vi "DMS_Multiplexer_Final.vi"() -> ()   [LabVIEW 2011]
uses:
  <vilib>/Instr/_visa.llb/VISA Configure Serial Port (Instr).vi
panel:
  out "error out":errorcluster
  in  "Dwell Time(s)":i32=20
  in  "No of Channels":i32=4
  in  "VISA resource name":refnum<visa-resource-name>="COM7"
  in  "Port B Read command\n(ASCII 'A'/41H)":string="Aÿ"
  out "USB Output String\n     (Bits 1-4)":string
  out "USB Port read status\n (Bits 8-5 = DIO, Bits 4-1 = Relays)":string
  out "Number":u32 format="%.0x"
  in  "Port B (Bits 1-8) Direction command\n (ASCII 'B'/42H)\n(0=output/1=input)":string="Bð"
  in  "Delay period \n(between channel activation)":dbl=20.0
  in  "Quit":bool
  # "USB4Mx (LV7.1 - Visa serial vi's)\n(8 bit (Port B) 4 output & 4 input channels)"
  # "Port Configuration/\nInitialisation characters"
  # "Relay control (Channels 1-4)"
  # "Port B Write command\n(ASCII 'C'/43H)"
  # "Voltage input channel status (Channels 8-5)"
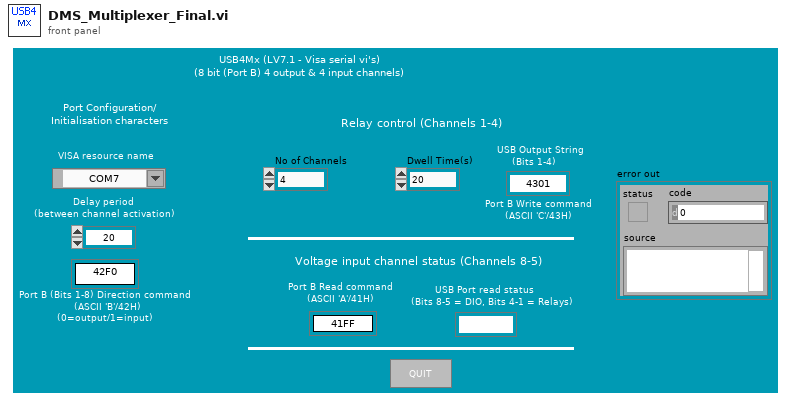
[diagram p1: front panel]
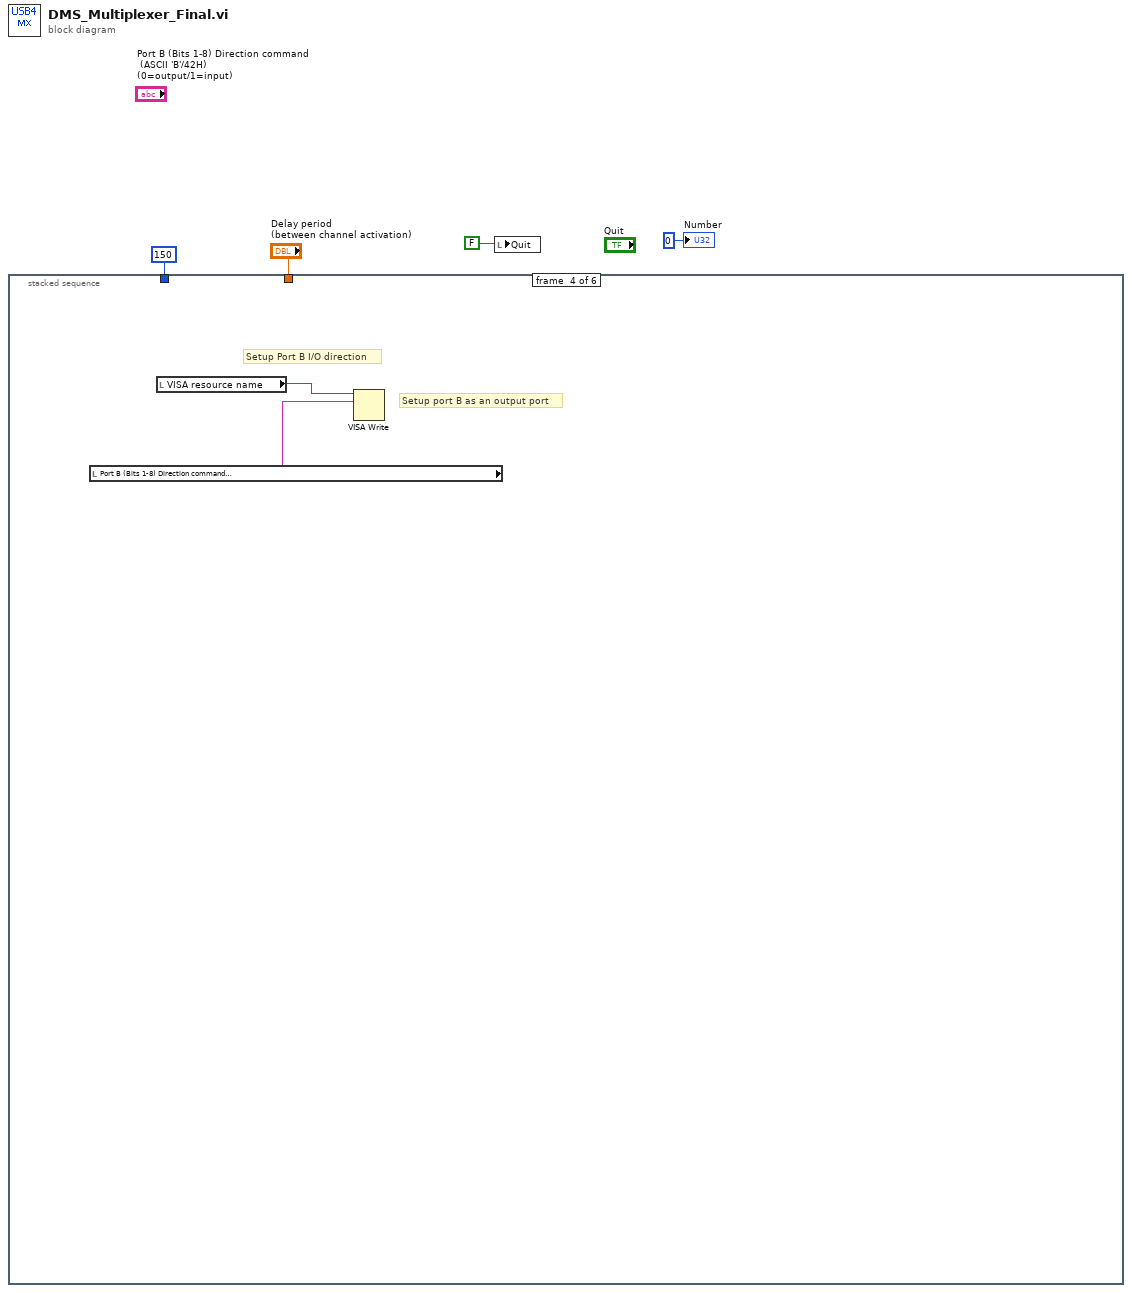
[diagram p0: block diagram]
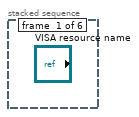
[diagram p2: hidden frame]
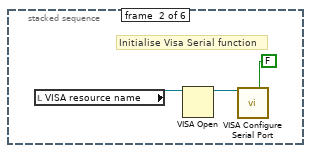
[diagram p3: hidden frame]
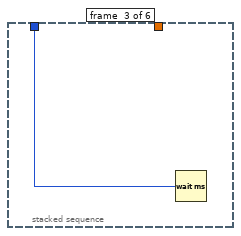
[diagram p4: hidden frame]
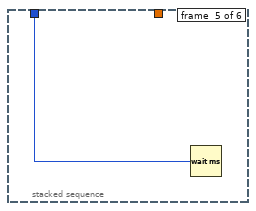
[diagram p5: hidden frame]
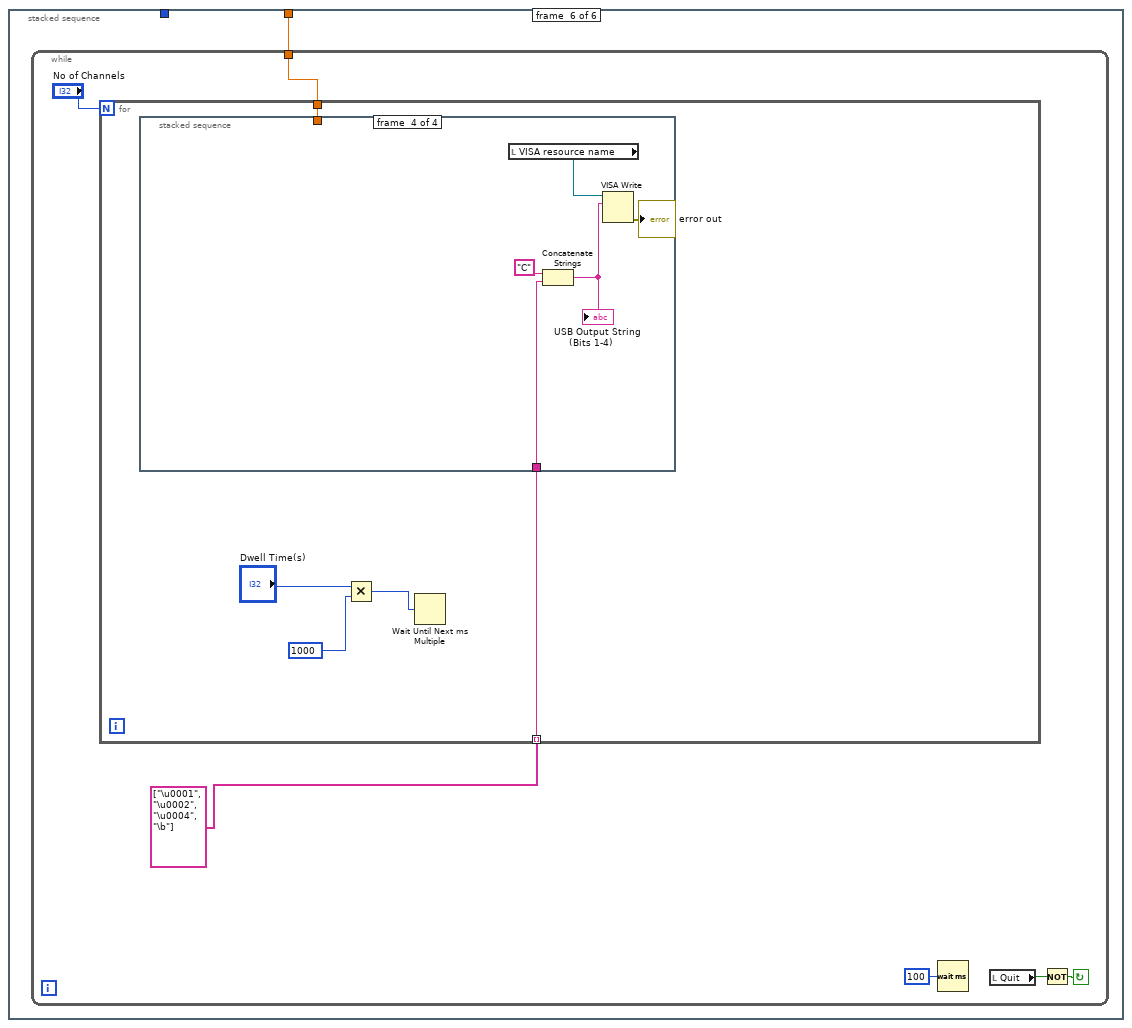
[diagram p6: hidden frame]
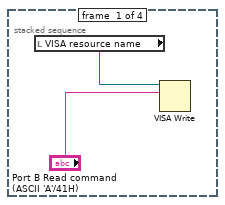
[diagram p7: hidden frame]
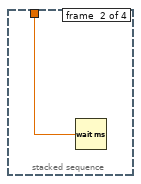
[diagram p8: hidden frame]
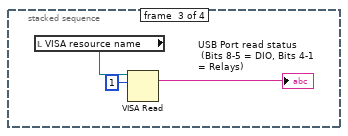
[diagram p9: hidden frame]
diagram:
  n1 = stacked-sequence {
    tunnel: 150 -> [_ _ w8 _ w11 _]
    tunnel: "Delay period \n(between channel activation)" -> [_ _ _ _ _ w12]
    frame #0 {
    }
    frame #1 {
      # "Initialise Visa Serial function"
      n2 = local read "VISA resource name"() -> (w5:refnum<visa-resource-name>)
      n3 = VISA Open(VISA resource name=w5) -> (VISA resource name=w6:refnum<visa-resource-name>)  [unwired: 4 in, 1 out]
      n4 = call-poly "VISA Configure Serial Port"("VISA resource name"=w6, "Enable Termination\nChar (T)"=FALSE ("Enable Termination\nChar (T)")) -> ()  [unwired: 12 in, 2 out]
    }
    frame #2 {
      n5 = Wait (ms)(milliseconds to wait=w8) -> ()  [unwired: 1 out]
    }
    frame #3 {
      # "Setup port B as an output port"
      # "Setup Port B I/O direction"
      n6 = local read "Port B (Bits 1-8) Direction command\n (ASCII 'B'/42H)\n(0=output/1=input)"() -> (w10:string)
      n7 = local read "VISA resource name"() -> (w9:refnum<visa-resource-name>)
      n8 = VISA Write(VISA resource name=w9, write buffer=w10) -> ()  [unwired: 1 in, 3 out]
    }
    frame #4 {
      n9 = Wait (ms)(milliseconds to wait=w11) -> ()  [unwired: 1 out]
    }
    frame #5 {
      n10 = while {
        tunnel: w12 -> [w15]
        stop <- w18 continue-if-true
        n11 = for {
          N: "No of Channels" -> [_]
          tunnel: w15 -> [w23]
          tunnel: string[] ["\u0001", "\u0002", "\u0004", "\b"] -> [w22] mode=indexing
          n12 = stacked-sequence {
            tunnel: w23 -> [_ w26 _ _]
            tunnel: w22 -> [_ _ _ w31]
            frame #0 {
              n13 = local read "VISA resource name"() -> (w24:refnum<visa-resource-name>)
              n14 = VISA Write(VISA resource name=w24, write buffer="Port B Read command\n(ASCII 'A'/41H)") -> ()  [unwired: 1 in, 3 out]
            }
            frame #1 {
              n15 = Wait (ms)(milliseconds to wait=w26) -> ()  [unwired: 1 out]
            }
            frame #2 {
              n16 = local read "VISA resource name"() -> (w28:refnum<visa-resource-name>)
              n17 = VISA Read(VISA resource name=w28, byte count=u32 1) -> (read buffer=→"USB Port read status\n (Bits 8-5 = DIO, Bits 4-1 = Relays)":string)  [unwired: 1 in, 3 out]
            }
            frame #3 {
              n18 = local read "VISA resource name"() -> (w32:refnum<visa-resource-name>)
              n19 = Concatenate Strings("C" ("Output string (hex)"), w31) -> (w33:string)
              "USB Output String\n     (Bits 1-4)" <- w33
              n20 = VISA Write(VISA resource name=w32, write buffer=w33) -> (error out=→"error out":errorcluster)  [unwired: 1 in, 2 out]
            }
          }
          n21 = Multiply(x="Dwell Time(s)", y=u32 1000 ("millisecond multiple")) -> (x*y=w19:u32)
          n22 = Wait Until Next ms Multiple(millisecond multiple=w19) -> ()  [unwired: 1 out]
        }
        n23 = Wait (ms)(milliseconds to wait=u32 100) -> ()  [unwired: 1 out]
        n24 = local read "Quit"() -> (w17:bool)
        n25 = Not(x=w17) -> (.not. x?=w18:bool)
      }
    }
  }
  n26 = local write "Quit"(FALSE ("Quit")) -> ()
  "Number" <- u32 0 ("Number")
